vi "Check Column Position.vi"(8 "error in":errorcluster, 10 "Coords":T2, 11 "Peer Review":refnum<class "Peer Review.lvclass">) -> (0 "error out":errorcluster, 2 "Cell Position":T1, 4 "Valid Position?":bool)   [LabVIEW 2020, in "Peer Review.lvclass"]
uses:
  Peer Review.lvclass
  <vilib>/Utility/miscctls.llb/LVPoint32TypeDef.ctl
  <vilib>/Utility/miscctls.llb/LVRowAndColumnTypeDef.ctl
  Peer Review.lvclass/Peer Review.ctl
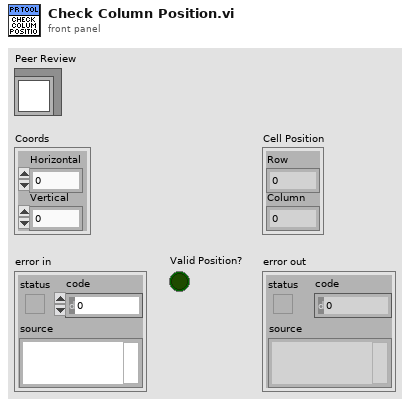
[diagram p1: front panel]
types:
  T1 = typedef "LVRowAndColumnTypeDef.ctl" = cluster{"Row":i32, "Column":i32}
  T2 = typedef "LVPoint32TypeDef.ctl" = cluster{"Horizontal":i32, "Vertical":i32}
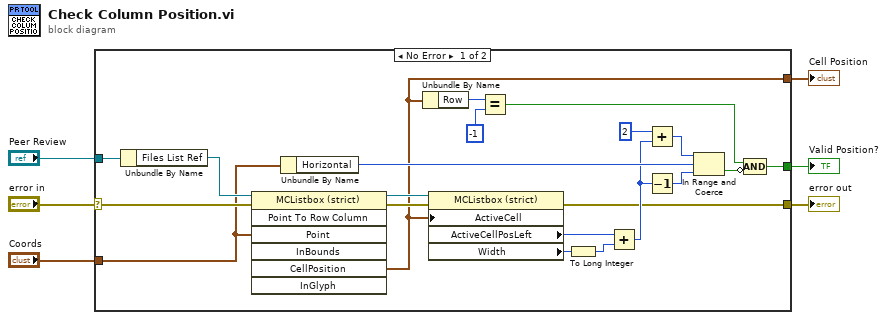
[diagram p0: block diagram]
diagram:
  n1 = case shown="No Error" "error in" {
    selector: "error in" -> [w24 w28]
    tunnel: [w13 w28] -> w5
    tunnel: "Peer Review" -> [w27 _]
    tunnel: "Coords" -> [w20 _]
    tunnel: [w8 _] -> w2
    tunnel: [w12 _] -> w1
    frame No Error {
      n2 = Unbundle By Name(w27) -> ("Files List Ref"=w22:refnum<vi>)
      n3 = invoke on="Invoke Node" class="MCListbox (strict)" method="Point To Row Column"(reference=w22, error in=w24, "Point"=w20) -> (reference out=w21:refnum<vi>, error out=w23:errorcluster, "CellPosition"=w12:T1)  [unwired: 4 in, 4 out]
      n4 = Unbundle By Name(w20) -> ("Horizontal"=w19:i32)
      n5 = Unbundle By Name(w12) -> ("Row"=w11:i32)
      n6 = property class="MCListbox (strict)"(reference=w21, error in=w23, "ActiveCell"=w12) -> (error out=w13:errorcluster, "ActiveCellPosLeft"=w26:i32, "Width"=w25:u32)  [unwired: 1 out]
      n7 = Equal?(x=w11, y=-1) -> (x = y?=w7:bool)
      n8 = To Long Integer(number=w25) -> (32bit integer=w17:i32)
      n9 = Add(x=w26, y=w17) -> (x+y=w16:i32)
      n10 = Add(x=2 ("y"), y=w16) -> (x+y=w14:i32)
      n11 = Decrement(x=w16) -> (x-1=w18:i32)
      n12 = In Range and Coerce(upper limit=w14, x=w19, lower limit=w18) -> (In Range?=w9:bool)  [unwired: 1 out]
      n13 = Compound Arithmetic op=AND(w7, invert w9) -> (w8:bool)
    }
    frame Error {
    }
  }
  "error out" <- w5
  "Valid Position?" <- w2
  "Cell Position" <- w1
